vi "Eagle RT Create 100 Points.vi"(4 "Radius B":fxp<+/-,10,10>=250.0, 6 "Radius A":fxp<+/-,10,10>=250.0, 9 "NumOfPoints":i32=100, 11 "Center":T1={"CX"=400.0, "CY"=300.0}) -> (2 "PY":i16[](array[numeric]), 3 "PX":i16[](array[numeric]))   [LabVIEW 2015]
panel:
  out "XY Graph":cluster{dbl[], dbl[]}(graph)
types:
  T1 = cluster{"CX":fxp<+/-,10,10>, "CY":fxp<+/-,10,10>}
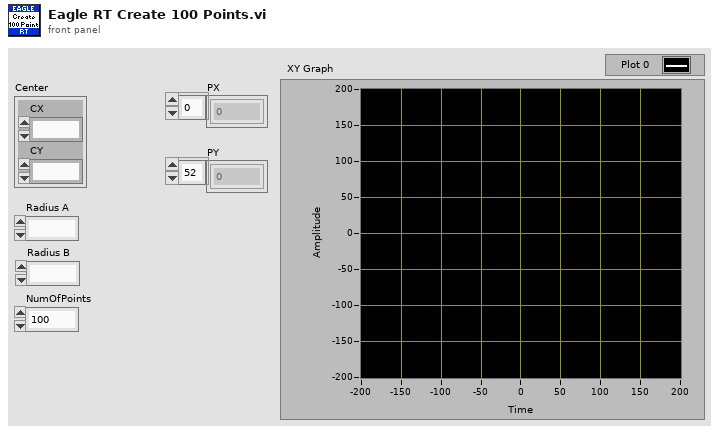
[diagram p1: front panel]
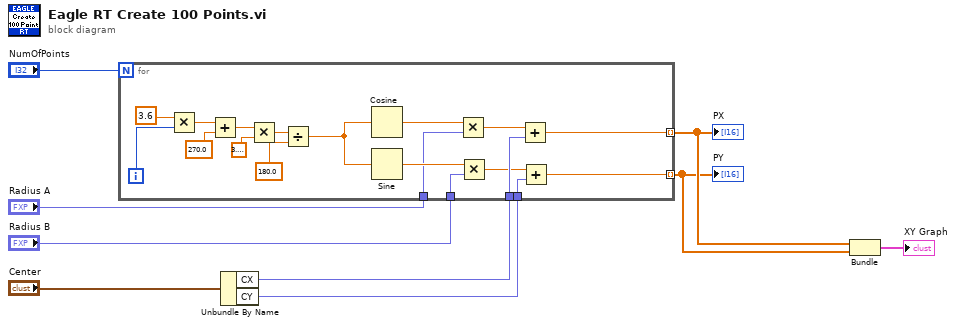
[diagram p0: block diagram]
diagram:
  n1 = Unbundle By Name("Center") -> ("CX"=w7:fxp<+/-,10,10>, "CY"=w6:fxp<+/-,10,10>)
  n2 = for {
    N: "NumOfPoints" -> [_]
    tunnel: w7 -> [w16]
    tunnel: w6 -> [w14]
    tunnel: [w11] -> w3 mode=indexing
    tunnel: [w10] -> w2 mode=indexing
    tunnel: "Radius B" -> [w13]
    tunnel: "Radius A" -> [w12]
    i -> [w27]
    n3 = Multiply(x=3.6, y=w27) -> (x*y=w26:dbl)
    n4 = Add(x=w26, y=270.0) -> (x+y=w21:dbl)
    n5 = Multiply(x=w21, y=3.141592653589793) -> (x*y=w23:dbl)
    n6 = Divide(x=w23, y=180.0) -> (x/y=w20:dbl)
    n7 = Cosine(x=w20) -> (cos(x)=w19:dbl)
    n8 = Sine(x=w20) -> (sin(x)=w18:dbl)
    n9 = Multiply(x=w19, y=w12) -> (x*y=w17:dbl)
    n10 = Multiply(x=w18, y=w13) -> (x*y=w15:dbl)
    n11 = Add(x=w17, y=w16) -> (x+y=w11:dbl)
    n12 = Add(x=w15, y=w14) -> (x+y=w10:dbl)
  }
  "PX" <- w3
  "PY" <- w2
  n13 = Bundle(w3, w2) -> (→"XY Graph":cluster{dbl[], dbl[]})  [unwired: 1 in]
